vi "Add.vi"(8 "error in (no error)":errorcluster, 11 "State Machine Data Class in":refnum<class "State Machine Data Class.lvclass">) -> (0 "error out":errorcluster, 3 "State Machine Data Class out":refnum<class "State Machine Data Class.lvclass">)   [LabVIEW 2020, in "Queue State Machine Lib.lvlib" / "State Machine Data Class.lvclass"]
uses:
  State Machine Data Class.lvclass
  State Machine Data Class.lvclass/State Machine Data Class.ctl
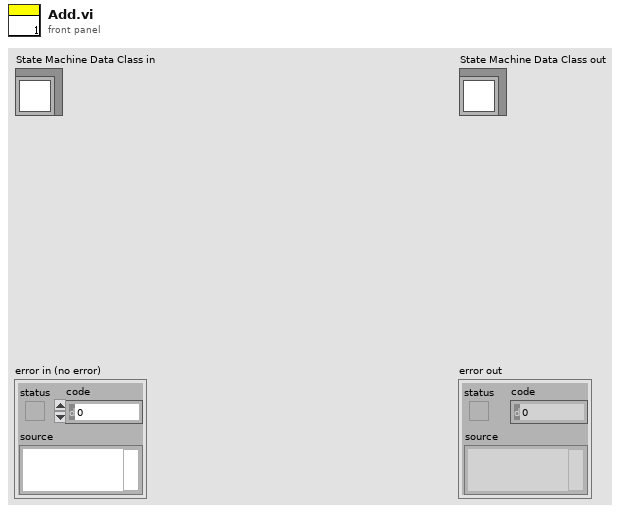
[diagram p1: front panel]
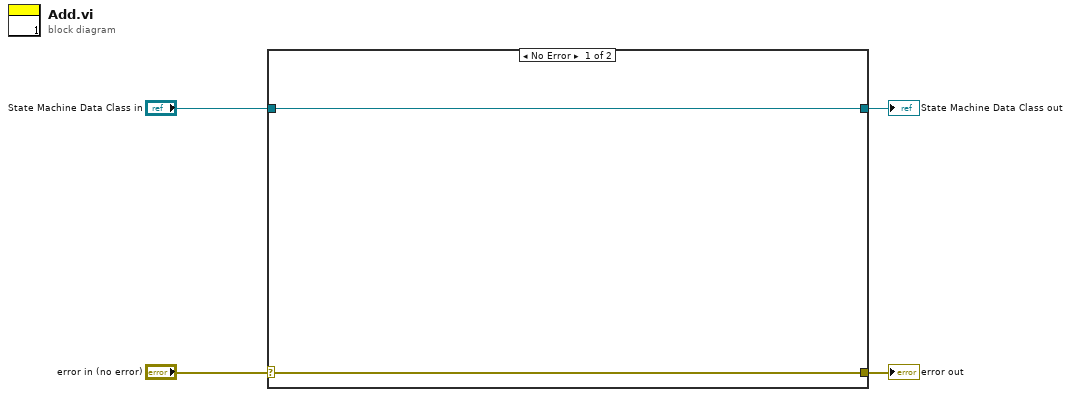
[diagram p0: block diagram]
diagram:
  n1 = case shown="No Error" "error in (no error)" {
    selector: "error in (no error)" -> [w5 w8]
    tunnel: [w5 w8] -> w3
    tunnel: [w6 w7] -> w1
    tunnel: "State Machine Data Class in" -> [w6 w7]
    frame No Error {
    }
    frame Error {
    }
  }
  "error out" <- w3
  "State Machine Data Class out" <- w1
